vi "Read.Lookup.vi"(8 "error in":errorcluster, 10 "Name":string, 11 "Plugin Data Access in":refnum<class "Plugin Data Access Engine.lvclass">) -> (0 "error out":errorcluster, 1 "Initial Values":dbl[](array[numeric]), 2 "Ref":T1, 3 "Plugin Data Access out":refnum<class "Plugin Data Access Engine.lvclass">)   [LabVIEW 2024, in "VS Plugin Data Access Engine.lvlib" / "Plugin Data Access Engine.lvclass"]
uses:
  Plugin Data Access Engine.lvclass
  Plugin Data Access Engine.lvclass/Plugin Data Access Engine.ctl
  Types/VS Channel Group Type.ctl
  Access Type Classes/Read/Read.lvclass
  Types/Read.DVR.ctl
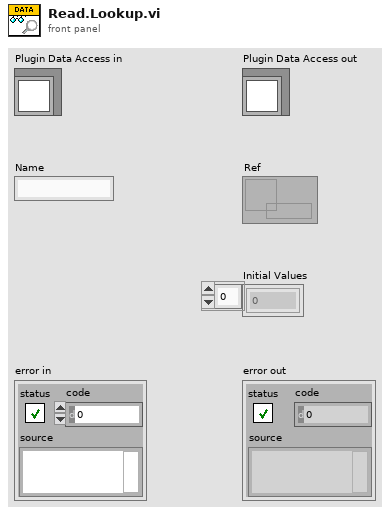
[diagram p1: front panel]
types:
  T1 = typedef "VS Plugin Data Access Engine.lvlib/Plugin Data Access Engine.lvclass/Read.DVR.ctl" = refnum<data-value>
  T2 = typedef "VS Plugin Data Access Engine.lvlib/Plugin Data Access Engine.lvclass/VS Channel Group Type.ctl" = enum16{"Output/Write", "Input/Read", "Input/ReadWrite"}
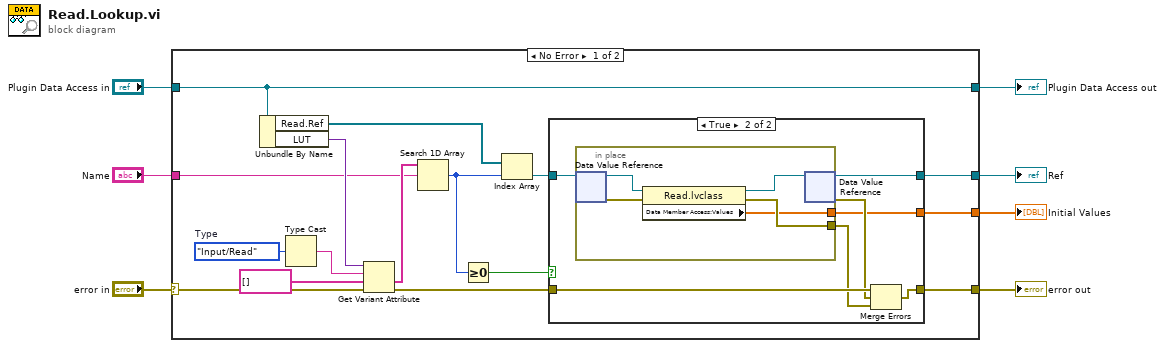
[diagram p0: block diagram]
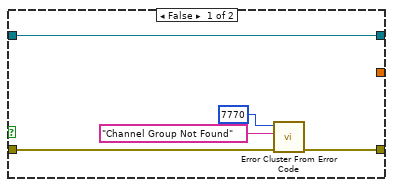
[diagram p2: hidden frame]
diagram:
  n1 = case shown="No Error" "error in" {
    selector: "error in" -> [w23 w42]
    tunnel: [w21 w42] -> w6
    tunnel: [w20 w41] -> w2
    tunnel: "Plugin Data Access in" -> [w20 w41]
    tunnel: "Name" -> [w12 _]
    tunnel: [w10 _] -> w1
    tunnel: [w8 _] -> w4
    frame No Error {
      w14 = VS_Channel_Group_Type."Input/Read"  # Type
      n2 = Unbundle By Name(w20) -> ("Read.Ref"=w15:refnum<data-value>[], "LUT"=w19:variant)
      n3 = Type Cast(x=w14) -> (*(type *) &x=w18:string)  [unwired: 1 in]
      n4 = Get Variant Attribute(Variant=w19, name=w18, default value (empty Variant)=string[] [], error in=w23) -> (value=w16:string[], error out=w22:errorcluster)  [unwired: 2 out]
      n5 = Search 1D Array(1D array=w16, element=w12) -> (index of element=w11:i32)  [unwired: 1 in]
      n6 = Greater Or Equal To 0?(x=w11) -> (x >= 0?=w13:bool)
      n7 = Index Array(array=w15, index=w11) -> (element=w9:refnum<data-value>)
      n8 = case shown="True" w13 {
        tunnel: w22 -> [w28 w35]
        tunnel: [w27 w34] -> w21
        tunnel: [w24 w30] -> w10
        tunnel: w9 -> [w24 w31]
        tunnel: [_ w29] -> w8
        frame False {
          n9 = call <vilib>:"Error Cluster From Error Code.vi"("error in (no error)"=w28, "error message (\"\")"="Channel Group Not Found" ("error message (\"\")"), "error code (0)"=7770) -> ("error out"=w27:errorcluster)  [unwired: 6 in]
        }
        frame True {
          n10 = in-place {
            in-place-border: [w36] -> w29
            in-place-border: [w39] -> w32
            n11 = in-place-dvr #1(w31) -> (w38:refnum<class "Read.lvclass">, w40:errorcluster)
            n12 = property class="Read.lvclass"(reference=w38, error in=w40) -> (reference out=w37:refnum<class "Read.lvclass">, error out=w39:errorcluster, "Data Member Access:Values"=w36:dbl[])
            n13 = in-place-dvr #1(w37) -> (w30:refnum<data-value>, w33:errorcluster)
          }
          n14 = Merge Errors(w35, w33, w32) -> (w34:errorcluster)
        }
      }
    }
    frame Error {
    }
  }
  "error out" <- w6
  "Plugin Data Access out" <- w2
  "Initial Values" <- w4
  "Ref" <- w1
